vi "Insert Item.vi"(8 "错误输入":errorcluster, 9 "Index":i32, 10 "Item":string, 11 "Listbox Ref":refnum<vi>) -> (0 "错误输出":errorcluster, 3 "Dup Listbox Ref":refnum<vi>)   [LabVIEW 2012, in "Listbox Tool.lvlib"]
uses:
  Listbox Tool.lvlib
  Custom Type/Read and Write Mode.ctl
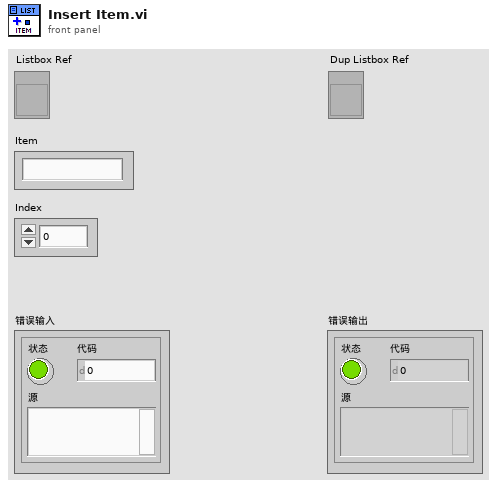
[diagram p1: front panel]
types:
  T1 = typedef "Listbox Tool.lvlib/Read and Write Mode.ctl" = enum16{"Read", "Write"}
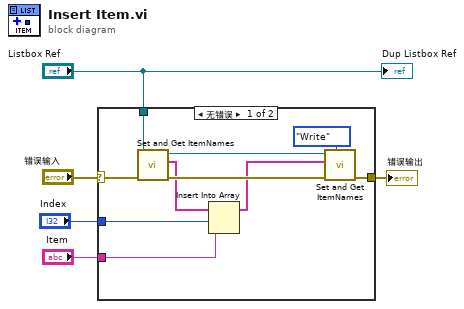
[diagram p0: block diagram]
diagram:
  n1 = case shown="无错误" "错误输入" {
    selector: "错误输入" -> [w15 w16]
    tunnel: "Listbox Ref" -> [w6 _]
    tunnel: "Item" -> [w8 _]
    tunnel: [w11 w16] -> w3
    tunnel: "Index" -> [w9 _]
    frame No Error {
      n2 = call "Set and Get ItemNames.vi"("错误输入"=w15, "Listbox Ref"=w6) -> ("错误输出"=w14:errorcluster, "ItemNames Out"=w10:string[], "Dup Listbox Ref"=w13:refnum<vi>)  [unwired: 7 in]
      n3 = Insert Into Array(array=w10, index=w9, new element=w8) -> (w7:string[])
      n4 = call "Set and Get ItemNames.vi"("Mode"=Read_and_Write_Mode."Write", "错误输入"=w14, "ItemNames In"=w7, "Listbox Ref"=w13) -> ("错误输出"=w11:errorcluster)  [unwired: 5 in, 2 out]
    }
    frame Error {
    }
  }
  "错误输出" <- w3
  "Dup Listbox Ref" <- "Listbox Ref"
